vi "Read RxRyZ limits.vi"(8 "error in (no error)":errorcluster, 11 "MotionSystem Configuration in":refnum<class "MotionSystem Configuration.lvclass">) -> (0 "error out":errorcluster, 2 "RxRyZ limits":T1 caption="Rx, Ry, Z limits" {"Z (um)"."soft limit max" format="%#_6f"; "Z (um)"."soft limit min" format="%#_6f"; "Ry (deg)"."soft limit max" format="%#_6f"; "Ry (deg)"."soft limit min" format="%#_6f"; "Rx (deg)"."soft limit max" format="%#_6f"; "Rx (deg)"."soft limit min" format="%#_6f"}, 3 "MotionSystem Configuration out":refnum<class "MotionSystem Configuration.lvclass">)   [LabVIEW 2016, in "MotionSystem.lvlib" / "MotionSystem Configuration.lvclass"]
uses:
  <userlib>/Common Components/Hardware/Abstract System/MotionSystem/MotionSystem Config/MotionSystem Configuration.lvclass
  <userlib>/Common Components/Hardware/Abstract System/MotionSystem/MotionSystem Config/RxRyZ Limits.ctl
  <userlib>/Common Components/Hardware/Abstract System/MotionSystem/MotionSystem Config/MotionSystem Configuration.lvclass/MotionSystem Configuration.ctl
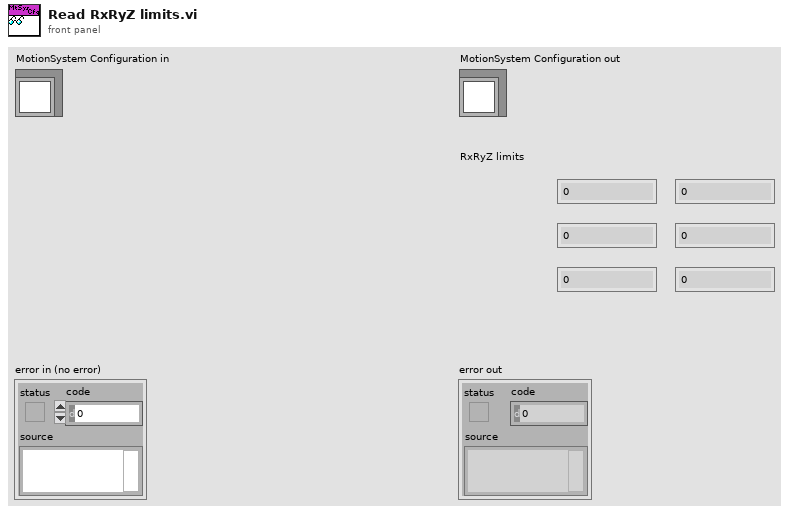
[diagram p1: front panel]
types:
  T1 = typedef "MotionSystem.lvlib/MotionSystem Configuration.lvclass/RxRyZ Limits.ctl" = cluster{"Rx (deg)":cluster{"label":string, "soft limit min":dbl, "soft limit max":dbl}, "Ry (deg)":cluster{"label":string, "soft limit min":dbl, "soft limit max":dbl}, "Z (um)":cluster{"label":string, "soft limit min":dbl, "soft limit max":dbl}}
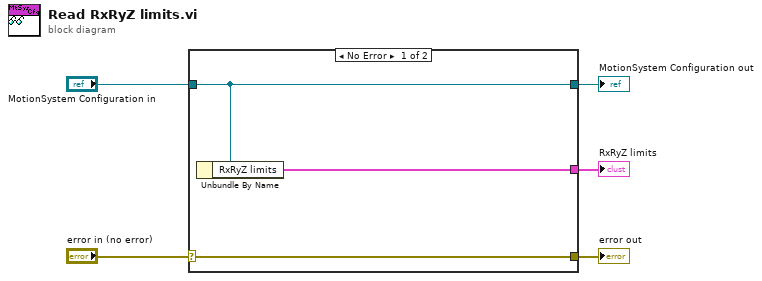
[diagram p0: block diagram]
diagram:
  n1 = case shown="No Error" "error in (no error)" {
    selector: "error in (no error)" -> [w8 w9]
    tunnel: [w8 w9] -> w4
    tunnel: [w7 w10] -> w2
    tunnel: "MotionSystem Configuration in" -> [w7 w10]
    tunnel: [w6 _] -> w1
    frame No Error {
      n2 = Unbundle By Name(w7) -> ("RxRyZ limits"=w6:T1)
    }
    frame Error {
    }
  }
  "error out" <- w4
  "MotionSystem Configuration out" <- w2
  "RxRyZ limits" <- w1
